vi "autoactions.vi"() -> ()   [LabVIEW 2012, in "MainProject.lvrbt"]
uses:
  MainProject.lvrbt
  <vilib>/NXT/Dual Mode Library/Waits/Wait_Num(msec).vi
  <vilib>/NXT/Hardware/Plugins/Tetrix DC Motor/TetrixDCMotorAddress.ctl
  <vilib>/NXT/LegoClasses/BrickReference/BrickReference.lvclass
  <vilib>/NXT/Subs/LVHSConnector.ctl
  <vilib>/NXT/NXTIO Xnodes/NXTIONodeSubVIs/TETRIX IO Check Battery.vi
  <vilib>/NXT/NXTIO Xnodes/NXTIOXNode/NXTIO.xnode
  <vilib>/NXT/NXTIO Xnodes/AddressXNode/NXTIOAddress.xnode
  <vilib>/NXT/NXTIO Xnodes/NXTIONodeSubVIs/TETRIX IO Stop DC Motors.vi
  Drivers/AutoControl3.ctl
  <vilib>/NXT/Block Support/NXT_InputPort.ctl
  <vilib>/NXT/HiTechnic/HiTechnic Controls/HiTechnic Port.ctl
  Drivers/AutoDriverControl.ctl
  <vilib>/NXT/Dual Mode Library/Waits/Wait_Num.vi
  <vilib>/NXT/Hardware/Plugins/Tetrix 180 deg Servo/Tetrix180ServoAddress.ctl
  <vilib>/NXT/NXTIO Xnodes/NXTIONodeSubVIs/TETRIX IO Move Servos.vi
  FTC 2012 - 2013/Controls/SpeedControl.ctl
  Drivers/LineCountColorCtl.ctl
  <vilib>/NXT/Dual Mode Library/Sound/Tone.vi
panel:
  out "Enabled 2":bool
  out "Line Color":string="Black"
  out "Sector (0-9)":i16
  in  "Dramatic Mode":bool
  out "Color":string="Black"
  out "Enabled":bool
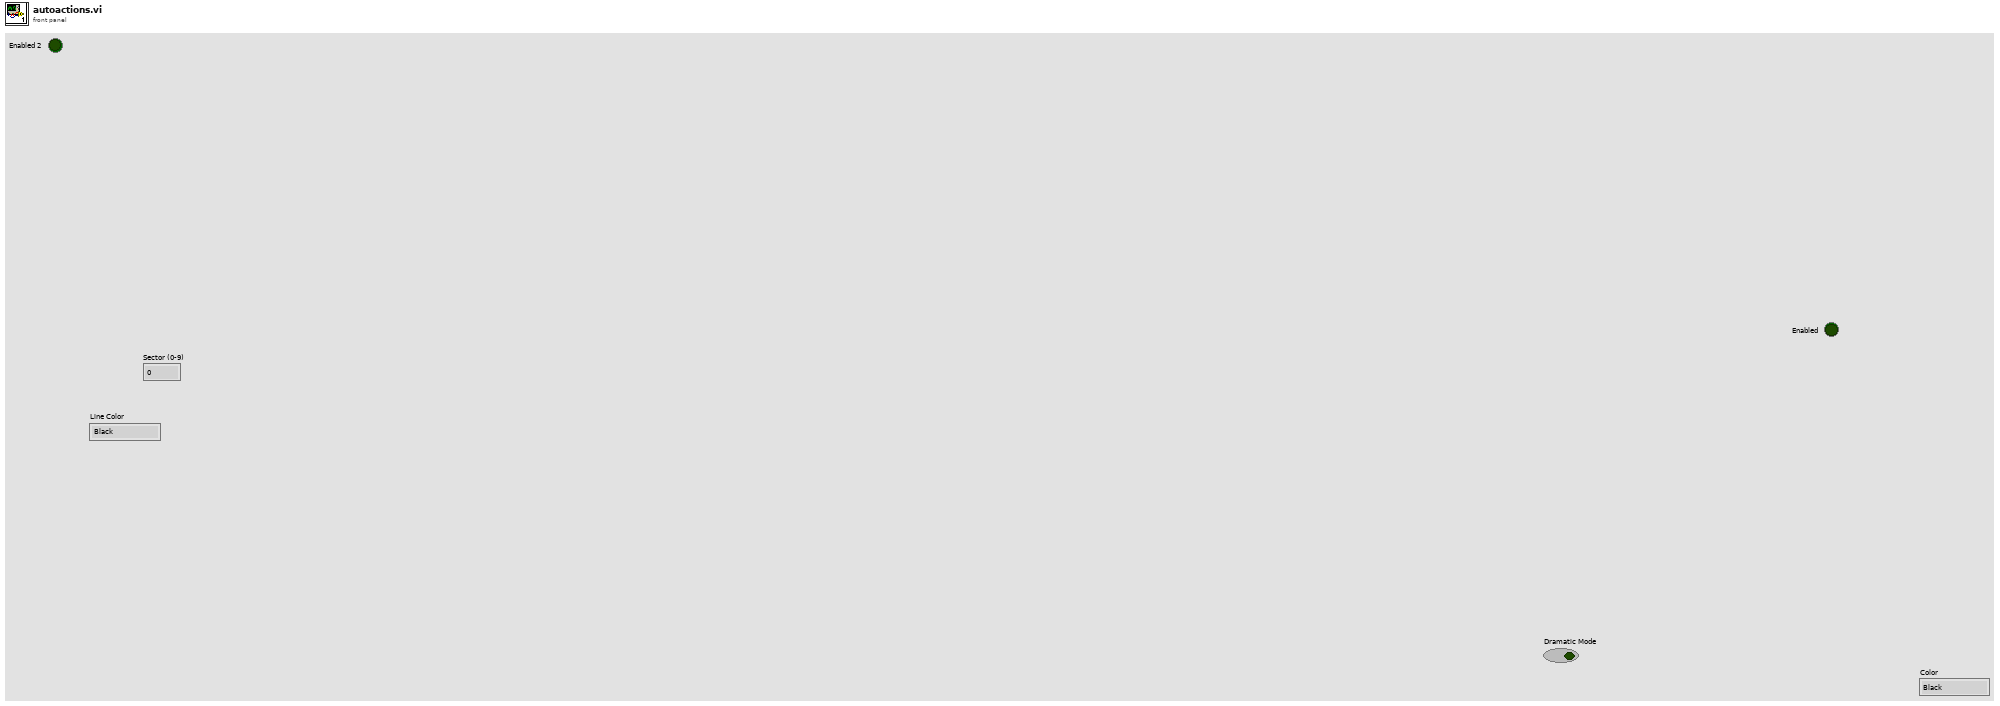
[diagram p1: front panel]
types:
  T1 = typedef "HiTechnic Port.ctl" = cluster{"Port":T2, "MUX Port":u8}
  T2 = typedef "NXT_InputPort.ctl" = u8
  T3 = typedef "TetrixDCMotorAddress.ctl" = i16
  T4 = typedef "LVHSConnector.ctl" = refnum<class "BrickReference.lvclass">
  T5 = typedef "Tetrix180ServoAddress.ctl" = i16
  T6 = typedef "AutoDriverControl.ctl" = enum16{"Init", "Forward", "Reverse", "Left", "Right", "Brake"}
  T7 = typedef "LineCountColorCtl.ctl" = enum16{"Init/Reset", "Check"}
  T8 = typedef "SpeedControl.ctl" = enum16{"Fast", "Medium", "Slow"}
  T9 = typedef "AutoControl3.ctl" = enum16{"FindIRBasket", "DropBLK", "DrvToEndOfBaskets", "DrvAroundBaskets", "AlignWithRamp", "ParkOnRamp", "Stop"}
  T10 = cluster{"Tetrix180Servo":T5, "Tetrix180Servo 2":T5, "Tetrix180Servo 3":T5, "Tetrix180Servo 4":T5}
  T11 = cluster{"Tetrix180Servo":T5, "Tetrix180Servo":T5, "Tetrix180Servo":T5, "Tetrix180Servo":T5}
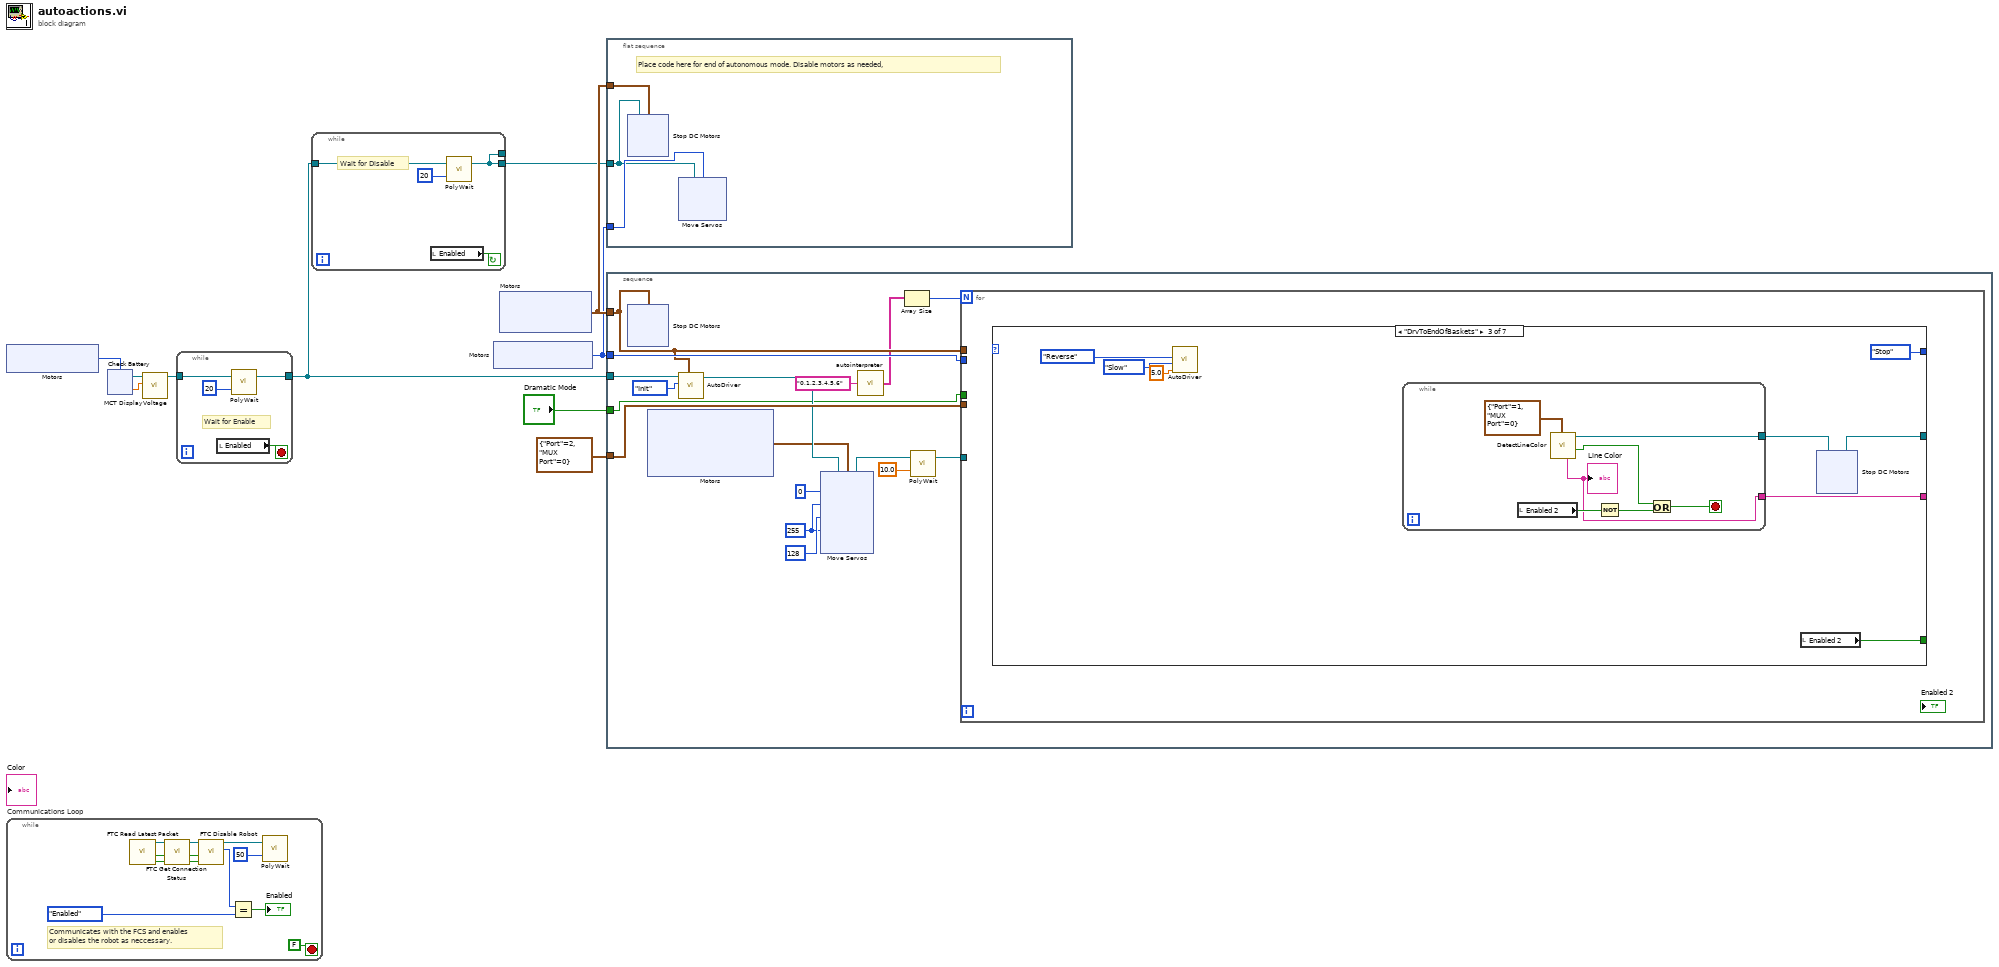
[diagram p0: block diagram]
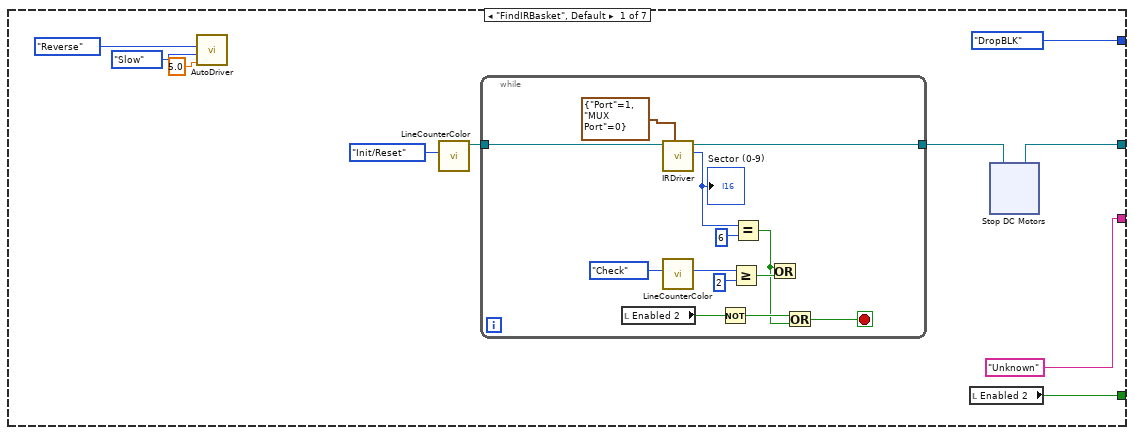
[diagram p2: hidden frame]
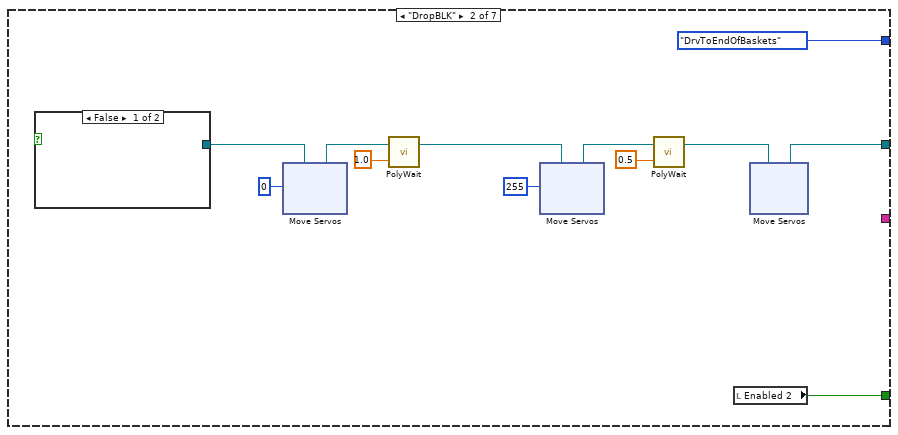
[diagram p3: hidden frame]
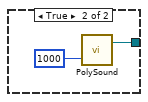
[diagram p4: hidden frame]
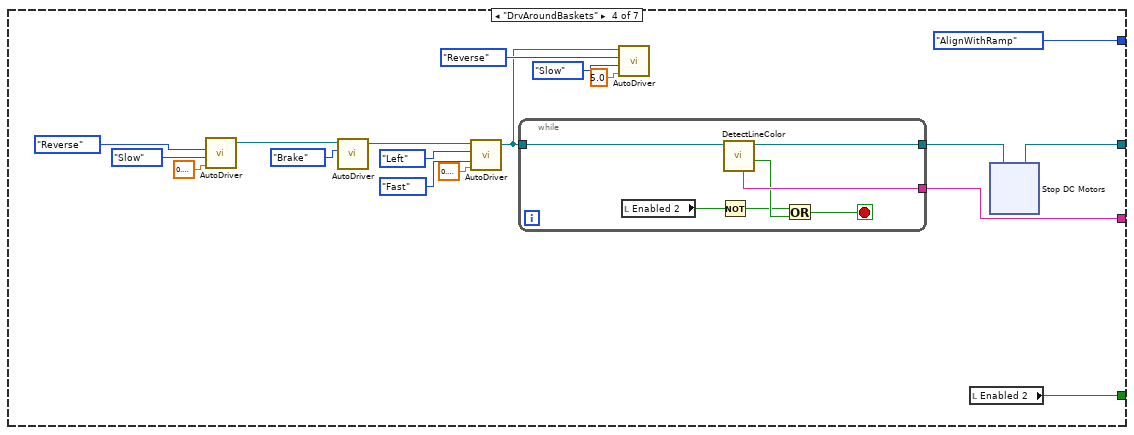
[diagram p5: hidden frame]
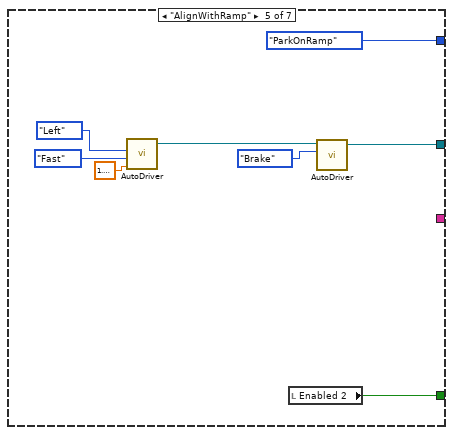
[diagram p6: hidden frame]
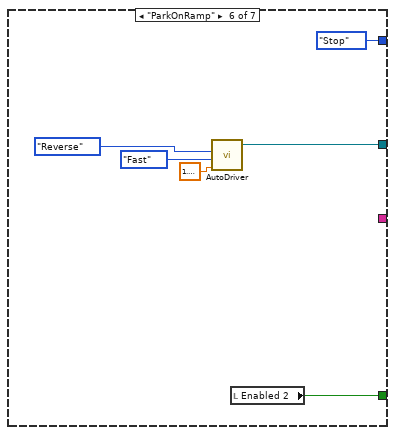
[diagram p7: hidden frame]
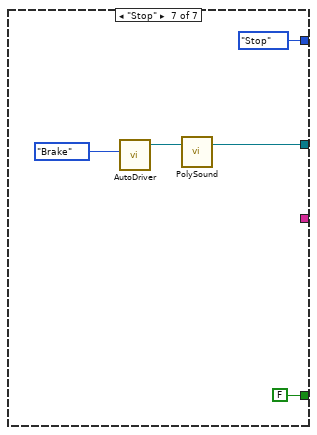
[diagram p8: hidden frame]
diagram:
  n1 = xnode "Motors"() -> ("Motor"=w5:T3)
  n2 = while "Communications Loop" {
    stop <- FALSE stop-if-true
    # "Communicates with the FCS and enables \nor disables the robot as neccessary."
    n3 = call <vilib>:"FTC Read Latest Packet.vi"() -> ("Packet Received?"=w20:bool, "Stopped?"=w19:bool, "NXT"=w22:T4)  [unwired: 6 in, 3 out]
    n4 = call <vilib>:"FTC Get Connection Status.vi"("Packet Received?"=w20, "Stopped?"=w19, "NXT"=w22) -> ("Online?"=w12:bool, "Stopped?"=w13:bool, "NXT"=w21:T4)  [unwired: 5 in]
    n5 = call <vilib>:"FTC Disable Robot.vi"("Online?"=w12, "Stopped?"=w13, "NXT"=w21) -> ("Enabled?"=w15:enum16{"Disabled", "Enabled"}, "NXT"=w17:T4)  [unwired: 3 in]
    n6 = Equal?(x=w15, y=enum16{"Disabled", "Enabled"}."Enabled") -> (x = y?=→"Enabled":bool)
    n7 = call-poly <vilib>:"PolyWait.vi"("Time (100 msec)"=u32 50 ("Time (msec)"), "NXT"=w17) -> ()  [unwired: 2 in, 1 out]
  }
  n8 = xnode "Check Battery"("Motors"=w5) -> ("Voltage 1"=w9:sgl, "NXT"=w10:T4)  [unwired: 1 in]
  n9 = call <vilib>:"MCT DisplayVoltage.vi"("Motor Voltage"=w9, "NXT"=w10) -> ("NXT"=w8:T4)  [unwired: 9 in]
  n10 = while {
    tunnel: [w25] -> w3
    tunnel: w8 -> [w23]
    stop <- w24 stop-if-true
    # "Wait for Enable"
    n11 = local read "Enabled"() -> (w24:bool)
    n12 = call-poly <vilib>:"PolyWait.vi"("Time (100 msec)"=u32 20 ("Time (msec)"), "NXT"=w23) -> ("NXT"=w25:T4)  [unwired: 2 in]
  }
  n13 = while {
    tunnel: [w27] -> _
    tunnel: w3 -> [w28]
    tunnel: [w27] -> w2
    stop <- w29 continue-if-true
    # "Wait for Disable"
    n14 = local read "Enabled"() -> (w29:bool)
    n15 = call-poly <vilib>:"PolyWait.vi"("Time (100 msec)"=u32 20 ("Time (msec)"), "NXT"=w28) -> ("NXT"=w27:T4)  [unwired: 2 in]
  }
  n16 = xnode "Motors"() -> ("Motor"=w4:T5)
  n17 = xnode "Motors"() -> ("Motor"=w7:cluster{"TetrixDCMotor":T3, "TetrixDCMotor":T3})
  n18 = flat-sequence {
    tunnel: w7 -> [w32]
    tunnel: w4 -> [w33]
    tunnel: w2 -> [w31]
    frame #0 {
      # "Place code here for end of autonomous mode. Disable motors as needed,"
      n19 = xnode "Stop DC Motors"("Motors"=w32, "NXT"=w31) -> ()  [unwired: 1 out]
      n20 = xnode "Move Servos"("Servos"=w33, "NXT"=w31) -> ()  [unwired: 1 in, 1 out]
    }
  }
  n21 = stacked-sequence {
    tunnel: w7 -> [w59]
    tunnel: w3 -> [w63]
    tunnel: T1 {"Port"=2, "MUX Port"=0} ("Port/MUX") -> [w64]
    tunnel: w4 -> [w60]
    tunnel: "Dramatic Mode" -> [w51]
    frame #0 {
      w54 = u8 255 ("Position 2")
      n22 = xnode "Stop DC Motors"("Motors"=w59) -> ()  [unwired: 1 in, 1 out]
      n23 = xnode "Motors"() -> ("Motor"=w57:T11)
      n24 = call "AutoDriver.vi"("NXT In"=w63, "Motors"=w59, "Direction"=AutoDriverControl."Init") -> ("NXT Out"=w62:T4)  [unwired: 5 in]
      n25 = xnode "Move Servos"("Position 4"=w54, "Position 3"=u8 128 ("Position 5"), "Position 2"=w54, "Position 1"=u8 0, "Servos"=w57, "NXT"=w62) -> ("NXT"=w58:T4)
      n26 = call "autointerpreter.vi"("String"="0,1,2,3,4,5,6") -> ("array"=w50:string[])
      n27 = Array Size(array=w50) -> (size(s)=w49:i32)
      n28 = call-poly <vilib>:"PolyWait.vi"("Time (1 sec)"=sgl 10.0, "NXT"=w58) -> ("NXT"=w53:T4)  [unwired: 2 in]
      n29 = for {
        N: w49 -> [_]
        tunnel: w59 -> [_]
        tunnel: w53 -> [_]
        tunnel: w64 -> [_]
        tunnel: w60 -> [_]
        tunnel: w51 -> [_]
        n30 = case shown="\"DrvToEndOfBaskets\"" {
          selector: _ -> [_ _ _ _ _ _ _]
          tunnel: [AutoControl3."DropBLK" AutoControl3."DrvToEndOfBaskets" AutoControl3."Stop" AutoControl3."AlignWithRamp" AutoControl3."ParkOnRamp" AutoControl3."Stop" AutoControl3."Stop"] -> _
          tunnel: [w68 w99 w136 w158 w185 w193 FALSE] -> _
          tunnel: ["Unknown" ("Color") _ w130 w159 _ _ _] -> _
          tunnel: [w67 w98 w131 w152 w184 w192 w198] -> _
          frame "FindIRBasket", Default {
            n31 = call "AutoDriver.vi"("Direction"=AutoDriverControl."Reverse", "Speed"=SpeedControl."Slow", "Time (1 sec)"=sgl 5.0) -> ()  [unwired: 5 in, 1 out]
            n32 = call "LineCounterColor.vi"("Enum"=LineCountColorCtl."Init/Reset") -> ("NXT Out"=w66:T4)  [unwired: 9 in, 1 out]
            n33 = while {
              tunnel: w66 -> [w91]
              tunnel: [w88] -> w69
              stop <- w85 stop-if-true
              n34 = local read "Enabled 2"() -> (w86:bool)
              n35 = call "IRDriver.vi"("Port"=T1 {"Port"=1, "MUX Port"=0}, "NXT In"=w91) -> ("Sector (0-9)"=w93:i16, "NXT Out"=w88:T4)  [unwired: 8 in]
              "Sector (0-9)" <- w93
              n36 = call "LineCounterColor.vi"("Enum"=LineCountColorCtl."Check") -> ("Numeric"=w83:i16)  [unwired: 9 in, 1 out]
              n37 = Not(x=w86) -> (.not. x?=w84:bool)
              n38 = Greater Or Equal?(x=w83, y=i16 2) -> (x >= y?=w89:bool)
              n39 = Equal?(x=w93, y=i16 6) -> (x = y?=w82:bool)
              n40 = Or(x=w82, y=w89) -> ()  [unwired: 1 out]
              n41 = Or(x=w84, y=w82) -> (x .or. y?=w85:bool)
            }
            n42 = local read "Enabled 2"() -> (w68:bool)
            n43 = xnode "Stop DC Motors"("NXT"=w69) -> ("NXT"=w67:T4)  [unwired: 1 in]
          }
          frame "DropBLK" {
            n44 = case shown="False" {
              selector: _ -> [_ _]
              tunnel: [_ w107] -> w96
              frame False {
              }
              frame True {
                n45 = call-poly <vilib>:"PolySound.vi"("Duration (500 ms)"=u16 1000) -> ("NXT"=w107:T4)  [unwired: 3 in]
              }
            }
            n46 = xnode "Move Servos"("Position 1"=u8 0, "NXT"=w96) -> ("NXT"=w95:T4)  [unwired: 1 in]
            n47 = call-poly <vilib>:"PolyWait.vi"("Time (1 sec)"=sgl 1.0, "NXT"=w95) -> ("NXT"=w104:T4)  [unwired: 2 in]
            n48 = xnode "Move Servos"("Position 1"=u8 255, "NXT"=w104) -> ("NXT"=w103:T4)  [unwired: 1 in]
            n49 = call-poly <vilib>:"PolyWait.vi"("Time (1 sec)"=sgl 0.5, "NXT"=w103) -> ("NXT"=w100:T4)  [unwired: 2 in]
            n50 = local read "Enabled 2"() -> (w99:bool)
            n51 = xnode "Move Servos"("NXT"=w100) -> ("NXT"=w98:T4)  [unwired: 2 in]
          }
          frame "DrvToEndOfBaskets" {
            n52 = call "AutoDriver.vi"("Direction"=AutoDriverControl."Reverse", "Speed"=SpeedControl."Slow", "Time (1 sec)"=sgl 5.0) -> ()  [unwired: 5 in, 1 out]
            n53 = while {
              tunnel: [w150] -> w132
              tunnel: [w145] -> w130
              stop <- w148 stop-if-true
              n54 = local read "Enabled 2"() -> (w149:bool)
              n55 = call "DetectLineColor.vi"("Port/MUX"=T1 {"Port"=1, "MUX Port"=0} ("Port")) -> ("Detected Line?"=w146:bool, "NXT Out"=w150:T4, "Color"=w145:string)  [unwired: 8 in]
              "Line Color" <- w145
              n56 = Not(x=w149) -> (.not. x?=w147:bool)
              n57 = Or(x=w146, y=w147) -> (x .or. y?=w148:bool)
            }
            n58 = local read "Enabled 2"() -> (w136:bool)
            n59 = xnode "Stop DC Motors"("NXT"=w132) -> ("NXT"=w131:T4)  [unwired: 1 in]
          }
          frame "DrvAroundBaskets" {
            n60 = call "AutoDriver.vi"("Direction"=AutoDriverControl."Reverse", "Speed"=SpeedControl."Slow", "Time (1 sec)"=sgl 0.3) -> ("NXT Out"=w162:T4)  [unwired: 5 in]
            n61 = call "AutoDriver.vi"("NXT In"=w162, "Direction"=AutoDriverControl."Brake") -> ("NXT Out"=w161:T4)  [unwired: 6 in]
            n62 = call "AutoDriver.vi"("NXT In"=w161, "Direction"=AutoDriverControl."Left", "Speed"=SpeedControl."Fast", "Time (1 sec)"=sgl 0.8) -> ("NXT Out"=w154:T4)  [unwired: 4 in]
            n63 = while {
              tunnel: [w183] -> w159
              tunnel: [w182] -> w153
              tunnel: w154 -> [w177]
              stop <- w179 stop-if-true
              n64 = local read "Enabled 2"() -> (w181:bool)
              n65 = Not(x=w181) -> (.not. x?=w178:bool)
              n66 = call "DetectLineColor.vi"("NXT In"=w177) -> ("Detected Line?"=w180:bool, "NXT Out"=w182:T4, "Color"=w183:string)  [unwired: 8 in]
              n67 = Or(x=w178, y=w180) -> (x .or. y?=w179:bool)
            }
            n68 = call "AutoDriver.vi"("NXT In"=w154, "Direction"=AutoDriverControl."Reverse", "Speed"=SpeedControl."Slow", "Time (1 sec)"=sgl 5.0) -> ()  [unwired: 4 in, 1 out]
            n69 = local read "Enabled 2"() -> (w158:bool)
            n70 = xnode "Stop DC Motors"("NXT"=w153) -> ("NXT"=w152:T4)  [unwired: 1 in]
          }
          frame "AlignWithRamp" {
            n71 = call "AutoDriver.vi"("Direction"=AutoDriverControl."Left", "Speed"=SpeedControl."Fast", "Time (1 sec)"=sgl 1.1) -> ("NXT Out"=w187:T4)  [unwired: 5 in]
            n72 = local read "Enabled 2"() -> (w185:bool)
            n73 = call "AutoDriver.vi"("NXT In"=w187, "Direction"=AutoDriverControl."Brake") -> ("NXT Out"=w184:T4)  [unwired: 6 in]
          }
          frame "ParkOnRamp" {
            n74 = call "AutoDriver.vi"("Direction"=AutoDriverControl."Reverse", "Speed"=SpeedControl."Fast", "Time (1 sec)"=sgl 1.3) -> ("NXT Out"=w192:T4)  [unwired: 5 in]
            n75 = local read "Enabled 2"() -> (w193:bool)
          }
          frame "Stop" {
            n76 = call "AutoDriver.vi"("Direction"=AutoDriverControl."Brake") -> ("NXT Out"=w201:T4)  [unwired: 7 in]
            n77 = call-poly <vilib>:"PolySound.vi"("NXT"=w201) -> ("NXT"=w198:T4)  [unwired: 3 in]
          }
        }
      }
    }
  }
